vi "Write.vi"(8 "error in":errorcluster, 10 "data":bool[][](array[boolean])=[[TRUE, TRUE, FALSE, TRUE], [TRUE, TRUE, TRUE, FALSE], [TRUE, FALSE, FALSE, FALSE], [TRUE, FALSE, FALSE, FALSE], [TRUE, FALSE, FALSE, FALSE]], 11 "task/channels in":refnum<k21>[](array[refnum])) -> (0 "Array":errorcluster[](array[cluster]))   [LabVIEW 2022 SP3]
uses:
  <vilib>/DAQmx/write.llb/DAQmx Write (Digital 1D Bool NChan 1Samp 1Line).vi
  <vilib>/DAQmx/miscellaneous.llb/DAQmx Fill In Error Info.vi
  <vilib>/DAQmx/write.llb/DAQmx Write (Analog 1D DBL NChan 1Samp).vi
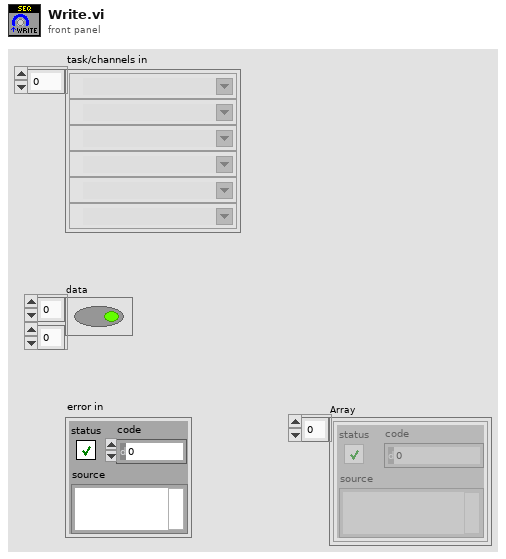
[diagram p1: front panel]
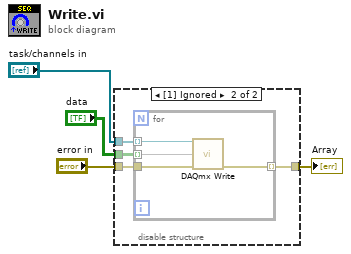
[diagram p0: block diagram]
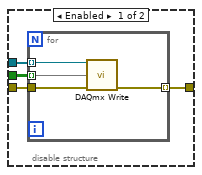
[diagram p2: hidden frame]
diagram:
  n1 = disable-structure shown="[1] Ignored" {
    disable-tunnel: "task/channels in" -> [w8 w16]
    disable-tunnel: "data" -> [w7 w15]
    disable-tunnel: "error in" -> [w6 w14]
    disable-tunnel: [w5 w13] -> w1
    frame Enabled {
      n2 = for {
        tunnel: w8 -> [w12] mode=indexing
        tunnel: w7 -> [w11] mode=indexing
        tunnel: [w10] -> w5 mode=indexing
        tunnel: w6 -> [w9]
        n3 = call-poly <vilib>:"DAQmx Write.vi"("task/channels in"=w12, "data"=w11, "error in"=w9) -> ("error out"=w10:errorcluster)  [unwired: 10 in, 2 out]
      }
    }
    frame Disabled {
      n4 = for {
        tunnel: w16 -> [w20] mode=indexing
        tunnel: w15 -> [w19] mode=indexing
        tunnel: [w18] -> w13 mode=indexing
        tunnel: w14 -> [w17]
        n5 = call-poly <vilib>:"DAQmx Write.vi"("task/channels in"=w20, "data"=w19, "error in"=w17) -> ("error out"=w18:errorcluster)  [unwired: 10 in, 2 out]
      }
    }
  }
  "Array" <- w1
